vi "Meas Write Samples Stream to MAT File.vi"(7 "is int16?":bool, 8 "error in":errorcluster, 9 "int32":i32[][](array[numeric]), 10 "int16":i16[][](array[numeric]), 11 "stream session in":T1) -> (0 "error out":errorcluster, 3 "stream session out":T1)   [LabVIEW 2020]
doc: "Writes samples to samples stream created by 'Meas Create Samples Stream File'. Input format flag 'is int16?' must match format of the opened stream. Function updates byte offset of the next sample every time based on the written data."
uses:
  Meas Samples Stream.ctl
  octave/mat/MAT Type Representation.ctl
  <vilib>/Utility/error.llb/Error Cluster From Error Code.vi
  <vilib>/ErrorRing/Error Ring.xnode
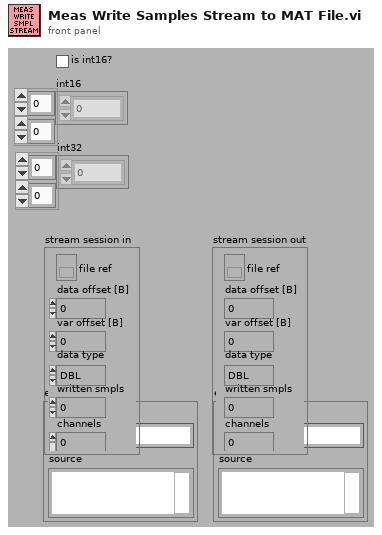
[diagram p1: front panel]
types:
  T1 = typedef "Meas Samples Stream.ctl" = cluster{"file ref":refnum<file>, "data offset [B]":i64, "var offset [B]":i64, "data type":T2, "written smpls":i64, "channels":i64}
  T2 = typedef "MAT Type Representation.ctl" = enum16{"DBL", "SGL", "I32", "I16", "U16", "U8", "CDB", "CSG", "STR"}
  T3 = enum16{"big-endian, network order", "native, host order", "little-endian"}
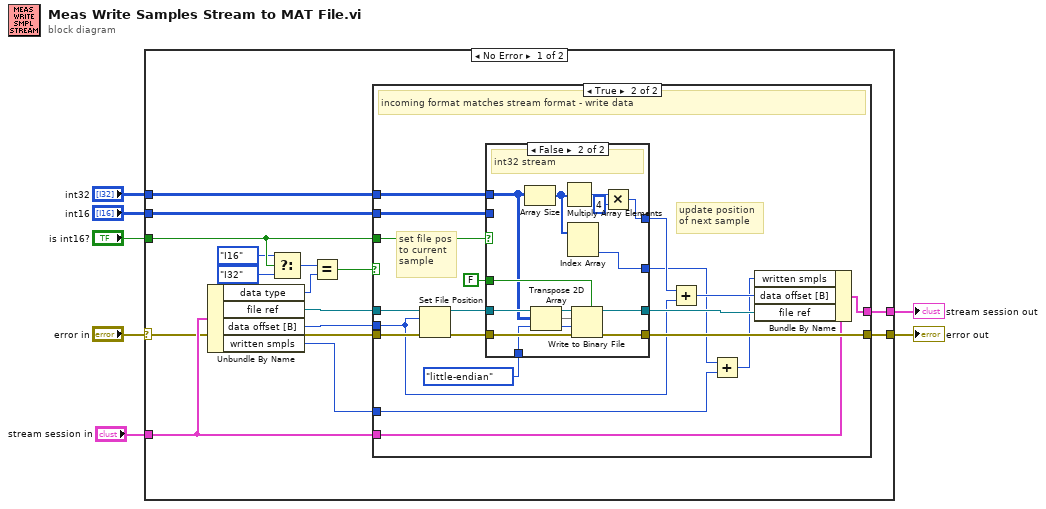
[diagram p0: block diagram]
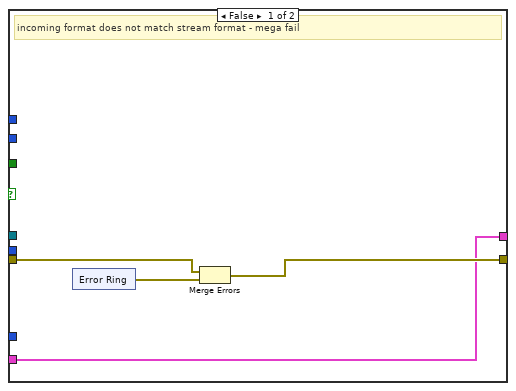
[diagram p2: hidden frame]
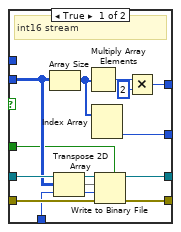
[diagram p3: hidden frame]
diagram:
  n1 = case shown="No Error" "error in" {
    selector: "error in" -> [w10 w78]
    tunnel: [w22 w78] -> w7
    tunnel: "int16" -> [w20 _]
    tunnel: "stream session in" -> [w19 w77]
    tunnel: [w18 w77] -> w4
    tunnel: "int32" -> [w17 _]
    tunnel: "is int16?" -> [w16 _]
    frame No Error {
      n2 = Unbundle By Name(w19) -> ("data type"=w12:T2, "file ref"=w21:refnum<file>, "data offset [B]"=w9:i64, "written smpls"=w8:i64)
      n3 = Select(t=MAT_Type_Representation."I16" ("data type"), s=w16, f=MAT_Type_Representation."I32" ("data type")) -> (s? t:f=w13:T2)
      n4 = Equal?(x=w13, y=w12) -> (x = y?=w11:bool)
      n5 = case shown="True" w11 {
        tunnel: w10 -> [w26 w41]
        tunnel: [w25 w50] -> w22
        tunnel: w21 -> [_ w38]
        tunnel: w20 -> [_ w48]
        tunnel: w19 -> [w24 w46]
        tunnel: [w24 w44] -> w18
        tunnel: w17 -> [_ w43]
        tunnel: w16 -> [_ w42]
        tunnel: w9 -> [_ w35]
        tunnel: w8 -> [_ w34]
        frame False {
          # "incoming format does not match stream format - mega fail"
          n6 = xnode "Error Ring"() -> ("error out"=w23:errorcluster)
          n7 = Merge Errors(w26, w23) -> (w25:errorcluster)
        }
        frame True {
          # "update position\nof next sample"
          # "set file pos\nto current\nsample"
          # "incoming format matches stream format - write data"
          n8 = Set File Position(offset (in bytes) (0)=w35, refnum=w38, error in=w41) -> (refnum out=w39:refnum<file>, error out=w40:errorcluster)  [unwired: 1 in]
          n9 = case shown="False" w42 {
            tunnel: w40 -> [w63 w76]
            tunnel: [w62 w75] -> w50
            tunnel: w39 -> [w61 w74]
            tunnel: T3."little-endian" ("byte order (0:big-endian, network order)") -> [w60 w73]
            tunnel: w48 -> [w58 _]
            tunnel: FALSE ("prepend array or string size? (T)") -> [w52 w72]
            tunnel: [w59 w71] -> w45
            tunnel: w43 -> [_ w68]
            tunnel: [w55 w67] -> w36
            tunnel: [w53 w65] -> w33
            frame True {
              # "int16 stream"
              n10 = Array Size(array=w58) -> (size(s)=w54:i32[])
              n11 = Transpose 2D Array(2D array=w58) -> (transposed array=w51:i16[][])
              n12 = Multiply Array Elements(1:w54) -> (0:w57:i32)
              n13 = Index Array(array=w54) -> (element #2=w53:i32)  [unwired: 2 in, 1 out]
              n14 = Write to Binary File(file (use dialog)=w61, data=w51, error in=w63, 5:w52, 9:w60) -> (refnum out=w59:refnum<file>, error out=w62:errorcluster)  [unwired: 1 in, 1 out]
              n15 = Multiply(x=w57, y=2) -> (x*y=w55:i32)
            }
            frame False {
              # "int32 stream"
              n16 = Array Size(array=w68) -> (size(s)=w66:i32[])
              n17 = Transpose 2D Array(2D array=w68) -> (transposed array=w64:i32[][])
              n18 = Multiply Array Elements(1:w66) -> (0:w70:i32)
              n19 = Index Array(array=w66) -> (element #2=w65:i32)  [unwired: 2 in, 1 out]
              n20 = Write to Binary File(file (use dialog)=w74, data=w64, error in=w76, 5:w72, 9:w73) -> (refnum out=w71:refnum<file>, error out=w75:errorcluster)  [unwired: 1 in, 1 out]
              n21 = Multiply(x=w70, y=4) -> (x*y=w67:i32)
            }
          }
          n22 = Add(x=w36, y=w35) -> (x+y=w37:i64)
          n23 = Add(x=w33, y=w34) -> (x+y=w32:i64)
          n24 = Bundle By Name(cluster=w46, "written smpls"=w32, "data offset [B]"=w37, "file ref"=w45) -> (w44:T1)
        }
      }
    }
    frame Error {
    }
  }
  "error out" <- w7
  "stream session out" <- w4
